vi "CallContextMenu.vi"(5 "CtrlRef":refnum<vi>, 6 "SubMenu":bool, 7 "User Event":refnum<user-event>, 8 "error in (no error)":errorcluster, 9 "Selected Tag":string, 10 "Selected Area":T1, 11 "Menu in":refnum<class "Menu.lvclass">) -> (0 "error out":errorcluster, 3 "Menu out":refnum<class "Menu.lvclass">)   [LabVIEW 2021, in "Menu.lvlib" / "Menu.lvclass"]
uses:
  Menu.lvclass
  SubMenu.vi
  <vilib>/Utility/error.llb/Error Cluster From Error Code.vi
  <vilib>/ErrorRing/Error Ring.xnode
  Menu.lvclass/Menu.ctl
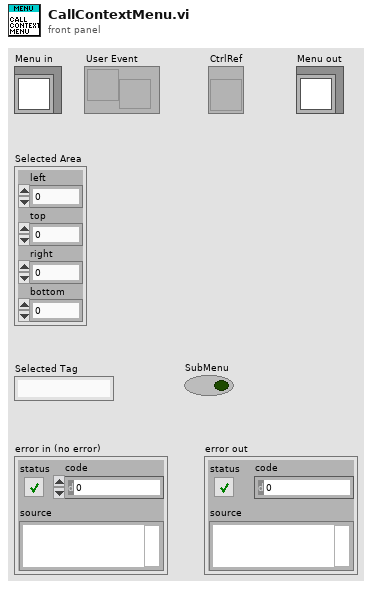
[diagram p1: front panel]
types:
  T1 = cluster{"left":i16, "top":i16, "right":i16, "bottom":i16}
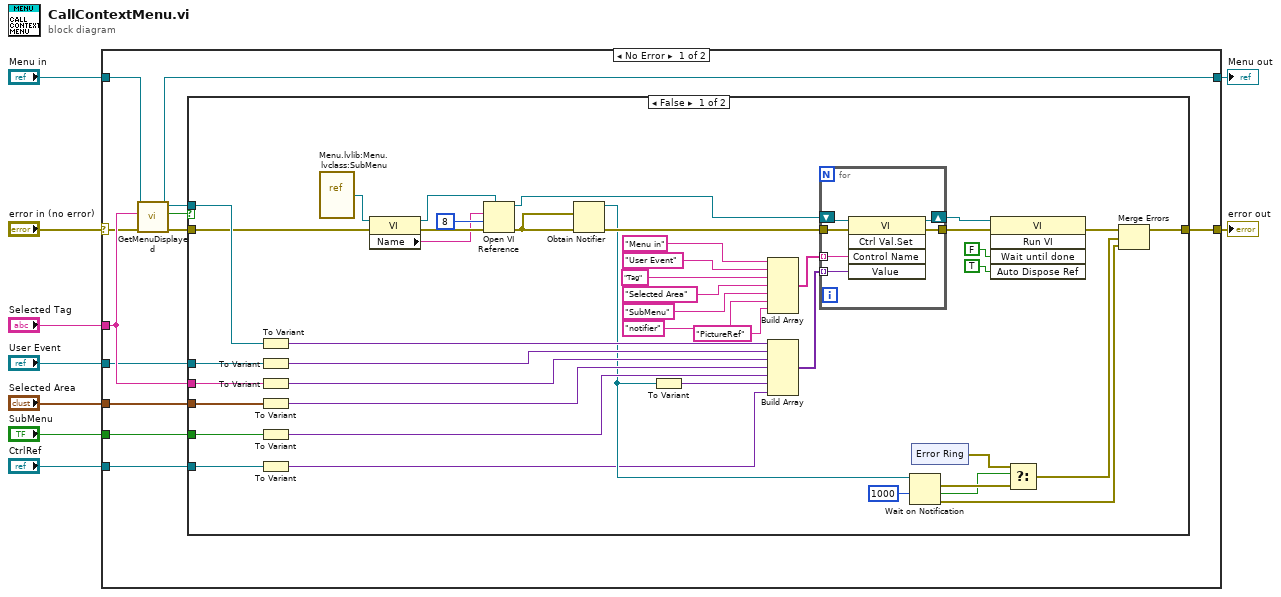
[diagram p0: block diagram]
diagram:
  n1 = case shown="No Error" "error in (no error)" {
    selector: "error in (no error)" -> [w14 w76]
    tunnel: [w20 w76] -> w9
    tunnel: "Selected Area" -> [w19 _]
    tunnel: "SubMenu" -> [w18 _]
    tunnel: "Menu in" -> [w17 w77]
    tunnel: [w16 w77] -> w5
    tunnel: "Selected Tag" -> [w15 _]
    tunnel: "User Event" -> [w12 _]
    tunnel: "CtrlRef" -> [w10 _]
    frame No Error {
      n2 = call "GetMenuDisplayed.vi"("error in (no error)"=w14, "Tag"=w15, "Menu in"=w17) -> ("error out"=w13:errorcluster, "Displayed?"=w11:bool, "Menu out"=w16:refnum<class "Menu.lvclass">)  [unwired: 6 in]
      n3 = case shown="False" w11 {
        tunnel: [w58 w75] -> w20
        tunnel: w19 -> [w64 _]
        tunnel: w18 -> [w63 _]
        tunnel: w16 -> [w62 _]
        tunnel: w15 -> [w61 _]
        tunnel: w13 -> [w60 w75]
        tunnel: w12 -> [w59 _]
        tunnel: w10 -> [w22 _]
        frame False {
          n4 = To Variant(anything=w62) -> (Variant=w43:variant)
          n5 = To Variant(anything=w59) -> (Variant=w41:variant)
          n6 = To Variant(anything=w61) -> (Variant=w42:variant)
          n7 = To Variant(anything=w64) -> (Variant=w40:variant)
          n8 = To Variant(anything=w63) -> (Variant=w39:variant)
          n9 = To Variant(anything=w22) -> (Variant=w21:variant)
          n10 = vi-ref "Menu.lvlib:Menu.lvclass:SubMenu.vi"() -> (w53:refnum<vi>)
          n11 = property class="VI"(reference=w53, error in=w60) -> (reference out=w56:refnum<vi>, error out=w57:errorcluster, "Name"=w54:string)
          n12 = Open VI Reference(type specifier VI Refnum (for type only)=w56, vi path=w54, options=8, error in (no error)=w57) -> (vi reference=w36:refnum<vi>, error out=w32:errorcluster)  [unwired: 2 in]
          n13 = Obtain Notifier(notification data type=w32, error in (no error)=w32) -> (notifier out=w31:refnum<notifier>, error out=w33:errorcluster)  [unwired: 2 in, 1 out]
          n14 = To Variant(anything=w31) -> (Variant=w34:variant)
          n15 = Build Array("Menu in" ("Control Name"), "User Event" ("Control Name"), "Tag" ("Control Name"), "Selected Area" ("Control Name"), "SubMenu" ("Control Name"), "notifier" ("Control Name"), "PictureRef") -> (w37:string[])
          n16 = Build Array(w43, w41, w42, w40, w39, w34, w21) -> (w38:variant[])
          n17 = for {
            tunnel: [w73] -> w49
            tunnel: w38 -> [w72] mode=indexing
            tunnel: w37 -> [w71] mode=indexing
            tunnel: w33 -> [w69]
            shift-right: [w74] -> w50
            shift-left: w36 -> [w70]
            n18 = invoke class="VI" method="Ctrl Val.Set"(reference=w70, error in=w69, "Control Name"=w71, "Value"=w72) -> (reference out=w74:refnum<vi>, error out=w73:errorcluster)  [unwired: 1 in, 3 out]
          }
          n19 = Wait on Notification(notifier=w31, timeout in ms (-1)=1000) -> (notification=w26:errorcluster, timed out?=w25:bool, error out=w29:errorcluster)  [unwired: 2 in, 1 out]
          n20 = xnode "Error Ring"() -> ("error out"=w24:errorcluster)
          n21 = invoke class="VI" method="Run VI"(reference=w50, error in=w49, "Wait until done"=FALSE ("Wait Until Done"), "Auto Dispose Ref"=TRUE ("Auto Dispose Reference")) -> (error out=w28:errorcluster)  [unwired: 1 in, 4 out]
          n22 = Select(t=w24, s=w25, f=w26) -> (s? t:f=w27:errorcluster)
          n23 = Merge Errors(w28, w27, w29) -> (w58:errorcluster)
        }
        frame True {
        }
      }
    }
    frame Error {
    }
  }
  "Menu out" <- w5
  "error out" <- w9
